vi "_shapiro2.vi"(0 "Bias_LO_equip":T4={"Node address"=19, "CAN Interface"="CAN0", "Cartridge band"=10, "Slave Node in"={"Address"=19, "Serial Number"=[16, -88, -112, 75, 1, 8, 0, 24]}, "ObjHandle out"=93192256, "POL"=1, "sb"=1, "GPIB_SM (SIS S,V)"="24", "GPIB_DMM (SIS I)"="22", "GPIB_SM (MAG I) "="25", "GPIB_SG(LO)"="19", "GPIB_PW (PAMP) "="6", "GPIB_TMP1(8ch)"="12", "GPIB_TMP2(2ch)  "="13", "WCA_avg"=10, "Rsen"=10.0, "BiasModule"=1, "LOModule "=2, "WCA_LO_FREQ_SET"={"YTO Low freq. [GHz]"=14.66, "YTO High freq. [GHz]"=17.5, "Kvco"=1, "Lock Pol."=0, "SET LO FREQ"=104.0, "Multiplier"=6.0, "YTO (HEX)"=3847, "YTO coarse( FREQ)"=17.328005, "NULL PLL INTEGRATOR"=FALSE}, "Res for"=0} {"Res for" items=["none", "series res", "parallel res"]; "WCA_LO_FREQ_SET"."YTO coarse( FREQ)" min=25 max=150 step=0.0001 format="%.3f"; "WCA_LO_FREQ_SET"."Multiplier" min=3 max=6 step=3; "WCA_LO_FREQ_SET"."SET LO FREQ" min=25 max=150 step=0.0001 format="%.3f"; "WCA_LO_FREQ_SET"."Lock Pol." items=["Lower", "Upper"]; "WCA_LO_FREQ_SET"."Kvco" items=["7.5MHz/V", "15MHz/V"]; "WCA_LO_FREQ_SET"."YTO High freq. [GHz]" format="%.3f"; "WCA_LO_FREQ_SET"."YTO Low freq. [GHz]" format="%.3f"; "LOModule" items=["Manual Gunn+PAMP"=0, "B10Lab LO"=1, "WCA LO"=2, ""=3, "YIG発信器"=4, "none"=99]; "BiasModule" items=["B10Lab Bias"=0, "WCA BiasModule"=1, "none"=99]; "Slave Node in"."Serial Number" format="%.0x"; "Slave Node in"."Address" format="%.0x"; "Cartridge band" max=10 step=1; "Node address" format="%.0x"}, 1 "Control":T2={"GPIB_ATT"="28", "6501Dev#"=1, "GPIB_SP"="18", "GPIB_PM"="13", "GPIB_DSA"="11", "GPIB_DMM (TPD)"="23", "GPIB_MPI"="COM5", "mortor設定"=[{"Axis"=0, "ID"=0, "HIspeed"=200.0, "LOspeed"=100.0, "ACCEL(ms)"=100.0, "Sratio"=50.0, "フリーラン\n"=FALSE, "文字列"="DSB HOT/COLD"}, {"Axis"=1, "ID"=0, "HIspeed"=4.0, "LOspeed"=4.0, "ACCEL(ms)"=100.0, "Sratio"=50.0, "フリーラン\n"=TRUE, "文字列"="SubMM Att"}, {"Axis"=0, "ID"=0, "HIspeed"=200.0, "LOspeed"=100.0, "ACCEL(ms)"=100.0, "Sratio"=50.0, "フリーラン\n"=FALSE, "文字列"="MPI Port1"}, {"Axis"=1, "ID"=0, "HIspeed"=200.0, "LOspeed"=100.0, "ACCEL(ms)"=100.0, "Sratio"=50.0, "フリーラン\n"=FALSE, "文字列"="MPI Port2"}, {"Axis"=1, "ID"=0, "HIspeed"=200.0, "LOspeed"=100.0, "ACCEL(ms)"=100.0, "Sratio"=50.0, "フリーラン\n"=TRUE, "文字列"="gainComp"}], "DATAパス"=path "L:/cartridge/assembly/SN03/03-13/110627_GUNNDSB_full_P0", "DBパス "=path "Z:/band10/Labview_ALMA/MIX95/test", "comment"="110627_gunndsbfull_P0", "ColdCarts"="003601", "Th"=299.0, "Tc"=83.0, "Set_SIS_volt"=2.1774193548387095, "Offset"=0.0, "control"=0, "FreqLO"=936.0, "Set_Mag_Cur"=9.671532846715328, "MPI offset(mm)"=23.166, "HOT/COLD"=0} {"HOT/COLD" items=["DSB", "SBR", "GainComp"]; "control" items=["CLOSE LOOP", "OPEN LOOP", "Not Control"]}, 2 "shapiro":T5={"start(mA)"=7.5, "stop(mA)"=12.5, "step(mA)"=0.1, "start(mV)"=1.2, "stop(mV)"=2.4, "step(mV)"=0.05, "file_name"="", "パス"=path "", "save?"=FALSE}, 3 "demag":T1={"Start(mA)"=50.0, "Time(ms)"=200.0, "step"=1.0}) -> (7 "min Mag current":dbl=9.299999999999994)   [LabVIEW 2017]
uses:
  __sub_vi/WCA_NAOJ_sub_vi/WCA_Global.vi
  <vilib>/express/express arith-compare/Formula/XNode/ExpressFormulaBlockNode.xnode
panel:
  out "setV  2":dbl=2.0500000000000003 format="%^#_3e"
  out "read V 2":dbl=1.9895172119140625
  out "read V":dbl=1.9895172119140625
  out "setV":dbl=2.0500000000000003 format="%^#_3e"
  in  "Time1":i32=1000
  in  "time0":i32=1000
  in  "set0?":bool=TRUE
  out "最終ｖ－P":cluster{"配列":dbl[], "配列 2":dbl[]}(graph)={"配列"=[1.1456298828125, 1.192474365234375, 1.2392425537109375, 1.2921142578125, 1.3437652587890625, 1.3919830322265625, 1.4446258544921875, 1.498565673828125, 1.551055908203125, 1.5949249267578125, 1.641693115234375, 1.691741943359375, 1.7388916015625, 1.7914581298828125, 1.841278076171875, 1.8906402587890625, 1.94244384765625, 1.9892120361328125, 2.0401763916015625, 2.0946502685546875, 2.142181396484375, 2.1912384033203125, 2.2409820556640625, 2.299041748046875, 2.3421478271484375], "配列 2"=[-30.6280724, -30.7126453, -30.6432113, -29.8285878, -28.8226745, -28.2742312, -27.7713224, -27.416188, -27.2844051, -27.2606276, -27.1514704, -26.9669342, -26.9316475, -26.9688126, -26.6291899, -25.4204539, -27.5721648, -25.6077726, -26.8063028, -27.3817095, -27.5837271, -27.7222411, -27.8415536, -28.2694503, -28.7533358]}
  out "error out":errorcluster caption="エラー出力"
  out "Link済み":bool=TRUE
  in  "i-vクラスタ":T3={"start(mV)"=1.2, "stop(mV)"=2.4, "step(mV)"=0.05, "file_name"="", "IF OFF/ON"=TRUE, "SAVE OFF/ON"=FALSE, "frq(GHz)"=8.0, "avg"=1, "Sweep回数 "=0, "VminfromSS"=0.05, "測定モード"=1, "V　opt"=0} {"測定モード" items=["電圧スイープ", "毎回HOT/COLD"]; "Sweep回数" items=["一回のみ", "Hot/Cold"]}
  out "初期値のV-P":cluster{dbl[], dbl[]}(graph)={[1.144561767578125, 1.1879730224609375, 1.2427520751953125, 1.2915802001953125, 1.34521484375, 1.3924407958984375, 1.4434051513671875, 1.4994049072265625, 1.5497589111328125, 1.5975189208984375, 1.6425323486328125, 1.693572998046875, 1.742706298828125, 1.7903900146484375, 1.838531494140625, 1.8914031982421875, 1.933746337890625, 1.9895172119140625, 2.041778564453125, 2.09136962890625, 2.1396636962890625, 2.1887969970703125, 2.2403717041015625, 2.2969818115234375, 2.3427581787109375], [-30.8304151, -30.6772316, -30.107581, -29.8432144, -27.7399153, -28.1617408, -27.8889748, -27.5394179, -26.7829628, -26.8468134, -26.4610859, -24.7404096, -23.8501166, -23.4218326, -23.1909815, -22.4041456, -26.7635773, -19.9675096, -20.681012, -21.9305003, -23.9269468, -27.6053273, -27.9912893, -28.0575443, -28.1897034]}
  out "min":dbl=-25.2940201 format="%^#_3e"
  out "Imag　vs P":cluster{dbl[], dbl[]}(graph)={[7.5, 7.6, 7.699999999999999, 7.799999999999999, 7.899999999999999, 7.999999999999998, 8.099999999999998, 8.199999999999998, 8.299999999999997, 8.399999999999997, 8.499999999999996, 8.599999999999996, 8.699999999999996, 8.799999999999995, 8.899999999999995, 8.999999999999995, 9.099999999999994, 9.199999999999994, 9.299999999999994, 9.399999999999993, 9.499999999999993, 9.599999999999993, 9.699999999999992, 9.799999999999992, 9.899999999999991, 9.999999999999991, 10.09999999999999, 10.19999999999999, 10.29999999999999, 10.39999999999999, 10.49999999999999, 10.599999999999989, 10.699999999999989, 10.799999999999988, 10.899999999999988, 10.999999999999988, 11.099999999999987, 11.199999999999987, 11.299999999999986, 11.399999999999986, 11.499999999999986, 11.599999999999985, 11.699999999999985, 11.799999999999985, 11.899999999999984, 11.999999999999984, 12.099999999999984, 12.199999999999983, 12.299999999999983, 12.399999999999983, 12.499999999999982], [-19.9638353, -20.1224192, -20.3203745, -20.461387, -20.6775476, -20.8219024, -20.9481227, -21.0140396, -21.0412557, -21.0582317, -21.1095669, -21.1470253, -21.2842083, -21.6610961, -22.0660132, -22.772983, -23.7101758, -24.7300495, -25.2940201, -24.7962579, -23.8748733, -22.8188748, -21.9031444, -21.2534559, -20.9269821, -20.7228013, -20.6284768, -20.5521107, -20.5344835, -20.5554763, -20.5479088, -20.6079808, -20.6594033, -20.7001155, -20.7420899, -20.7889111, -20.8004769, -20.844337, -20.9141659, -20.907771, -20.9407614, -20.9712207, -21.005632, -21.0478521, -21.0781252, -21.2327487, -21.243586, -21.3534511, -21.5174431, -21.7408682, -21.9673929]}
  # "LO freq. [GHz]"
  # "YTO LOW\n/High Freq."
  # "ZERO Intgrtr"
  # "Node Address"
  # "Serial Number"
  # "Magnet current"
  # "SIS Bias range"
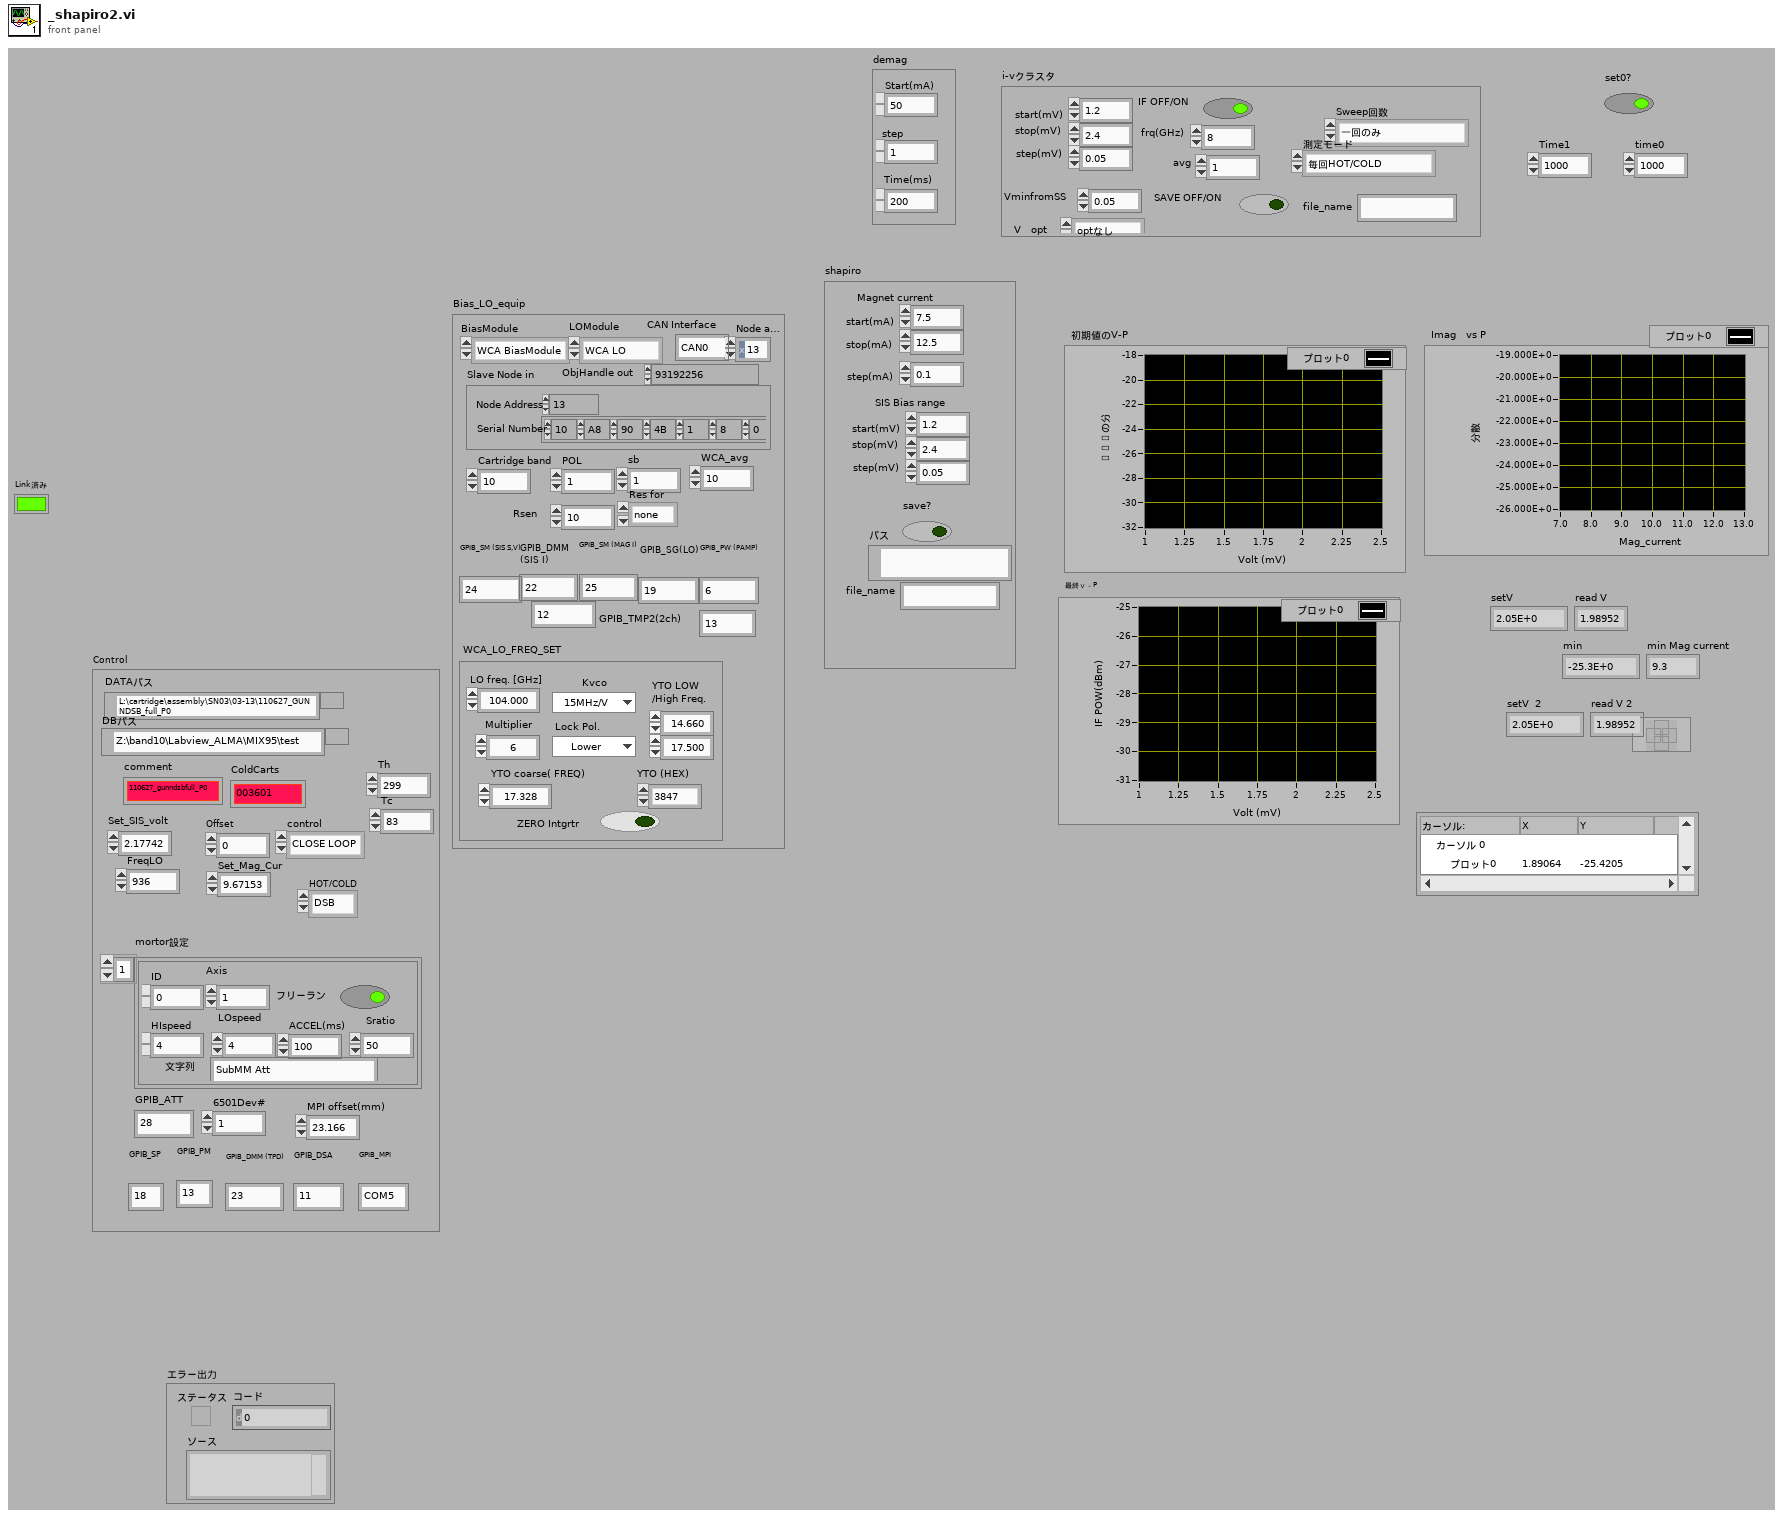
[diagram p1: front panel]
types:
  T1 = cluster{"Start(mA)":dbl, "Time(ms)":dbl, "step":dbl}
  T2 = cluster{"GPIB_ATT":string, "6501Dev#":i16, "GPIB_SP":string, "GPIB_PM":string, "GPIB_DSA":string, "GPIB_DMM (TPD)":string, "GPIB_MPI":string, "mortor設定":cluster{"Axis":i16, "ID":i16, "HIspeed":dbl, "LOspeed":dbl, "ACCEL(ms)":dbl, "Sratio":dbl, "フリーラン\n":bool, "文字列":string}[], "DATAパス":path, "DBパス ":path, "comment":string, "ColdCarts":string, "Th":dbl, "Tc":dbl, "Set_SIS_volt":dbl, "Offset":dbl, "control":u16, "FreqLO":dbl, "Set_Mag_Cur":dbl, "MPI offset(mm)":dbl, "HOT/COLD":u16}
  T3 = cluster{"start(mV)":dbl, "stop(mV)":dbl, "step(mV)":dbl, "file_name":string, "IF OFF/ON":bool, "SAVE OFF/ON":bool, "frq(GHz)":dbl, "avg":i32, "Sweep回数 ":u16, "VminfromSS":dbl, "測定モード":u16, "V　opt":u16}
  T4 = cluster{"Node address":u16, "CAN Interface":string, "Cartridge band":u32, "Slave Node in":cluster{"Address":i16, "Serial Number":i8[]}, "ObjHandle out":u32, "POL":u32, "sb":u32, "GPIB_SM (SIS S,V)":string, "GPIB_DMM (SIS I)":string, "GPIB_SM (MAG I) ":string, "GPIB_SG(LO)":string, "GPIB_PW (PAMP) ":string, "GPIB_TMP1(8ch)":string, "GPIB_TMP2(2ch)  ":string, "WCA_avg":i32, "Rsen":dbl, "BiasModule":u16, "LOModule ":u16, "WCA_LO_FREQ_SET":cluster{"YTO Low freq. [GHz]":sgl, "YTO High freq. [GHz]":sgl, "Kvco":u16, "Lock Pol.":u16, "SET LO FREQ":sgl, "Multiplier":sgl, "YTO (HEX)":u16, "YTO coarse( FREQ)":sgl, "NULL PLL INTEGRATOR":bool}, "Res for":u16}
  T5 = cluster{"start(mA)":dbl, "stop(mA)":dbl, "step(mA)":dbl, "start(mV)":dbl, "stop(mV)":dbl, "step(mV)":dbl, "file_name":string, "パス":path, "save?":bool}
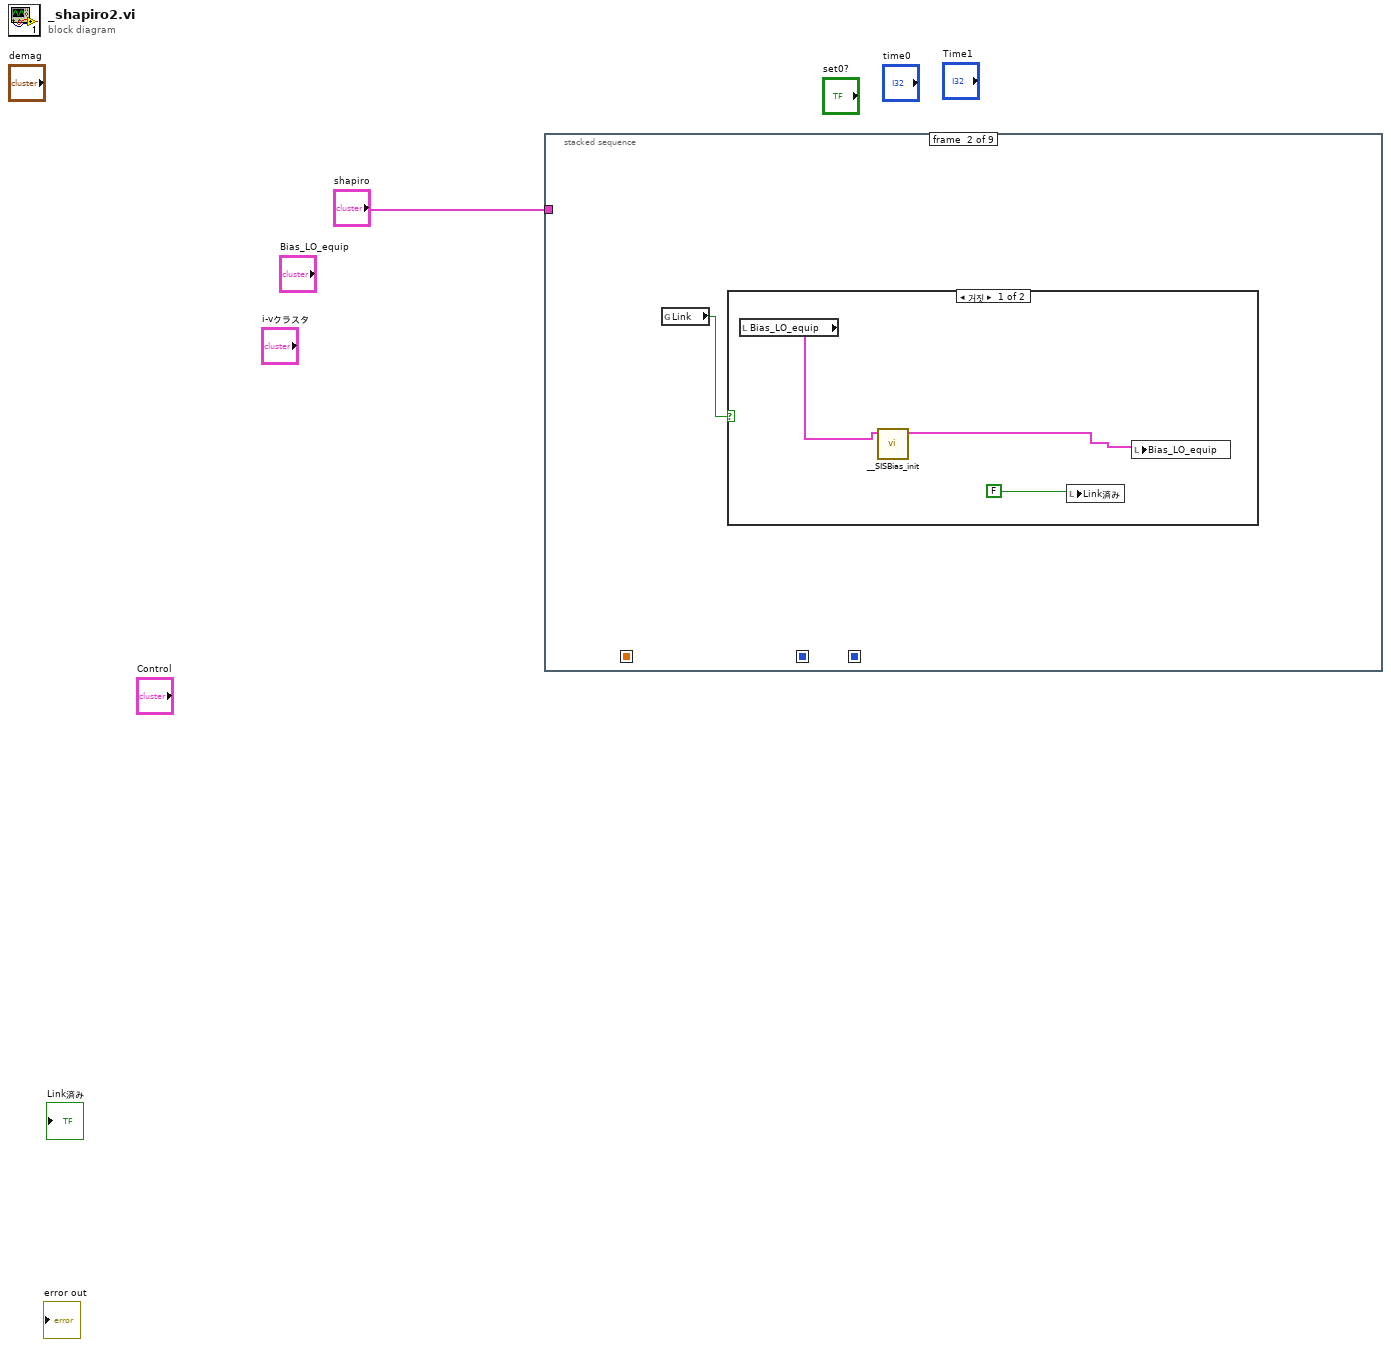
[diagram p0: block diagram]
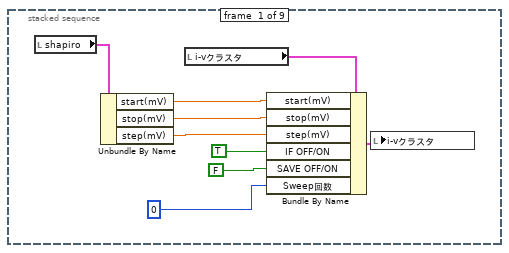
[diagram p2: hidden frame]
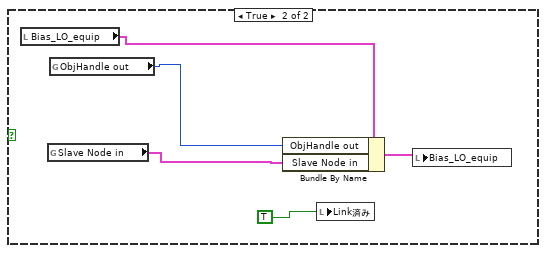
[diagram p3: hidden frame]
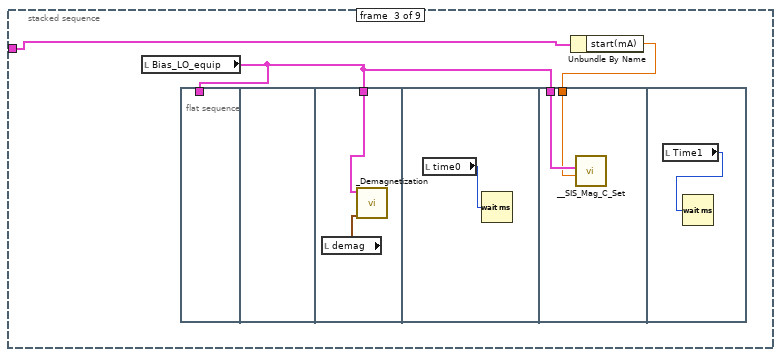
[diagram p4: hidden frame]
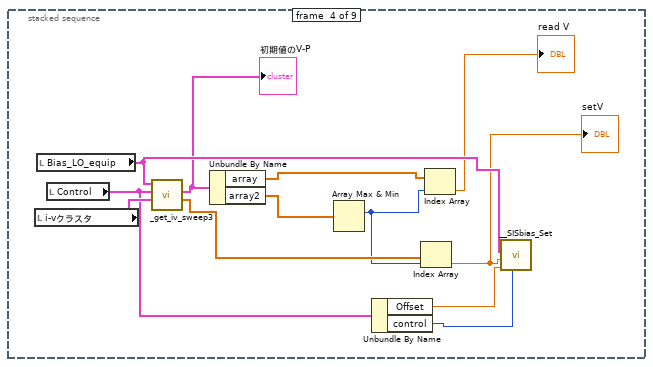
[diagram p5: hidden frame]
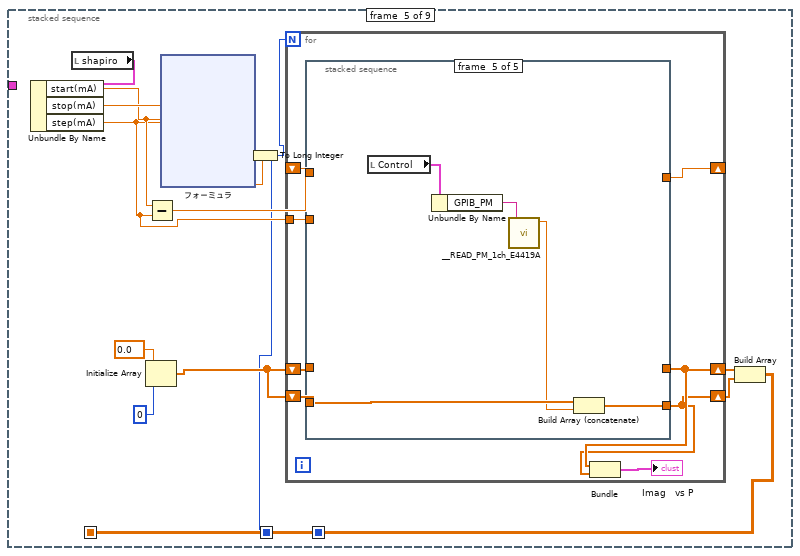
[diagram p6: hidden frame]
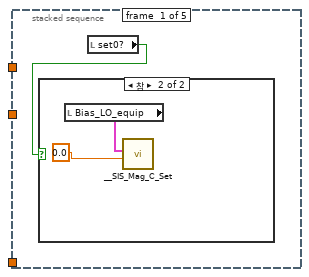
[diagram p7: hidden frame]
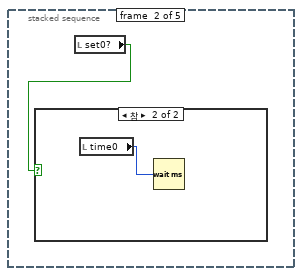
[diagram p9: hidden frame]
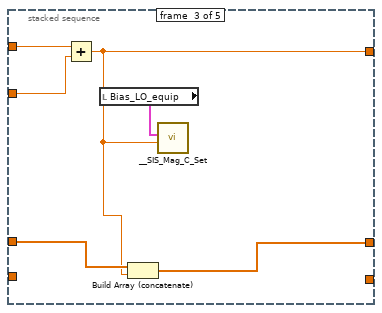
[diagram p11: hidden frame]
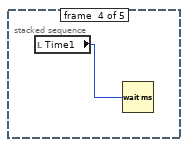
[diagram p12: hidden frame]
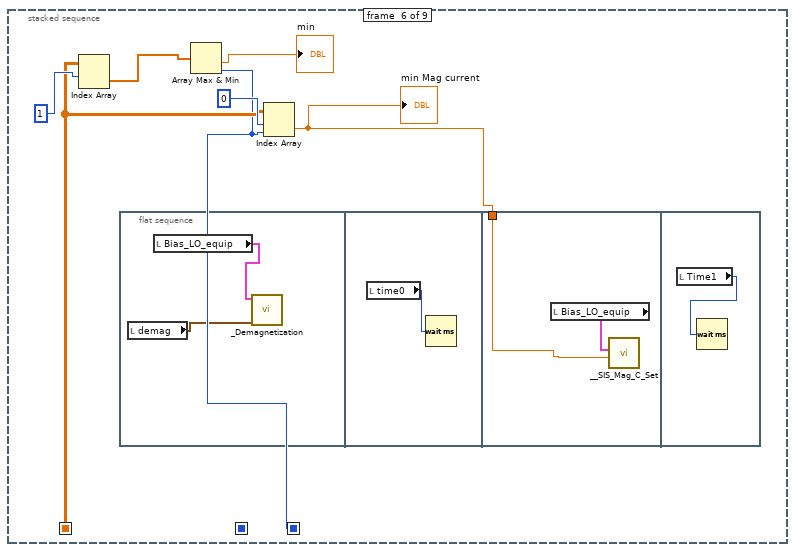
[diagram p13: hidden frame]
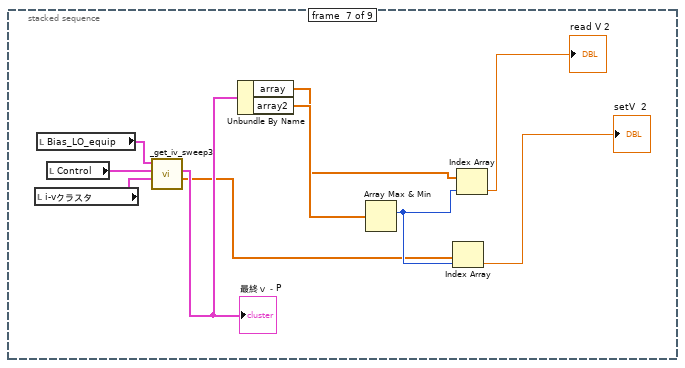
[diagram p14: hidden frame]
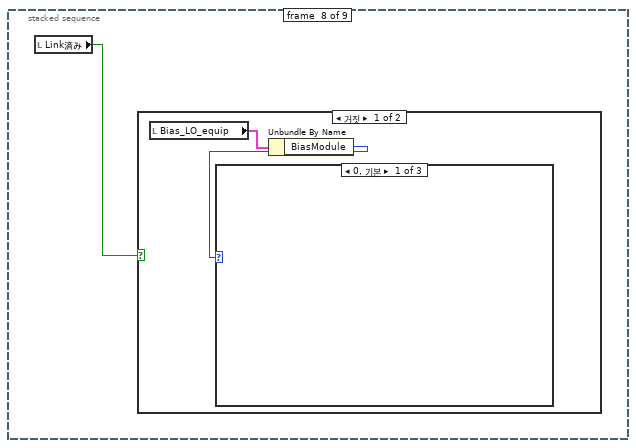
[diagram p15: hidden frame]
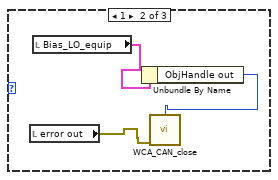
[diagram p16: hidden frame]
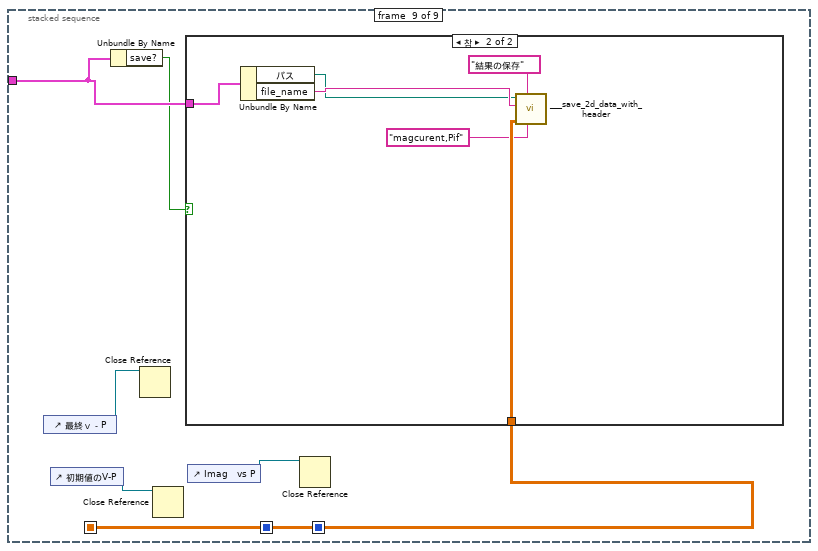
[diagram p19: hidden frame]
diagram:
  n1 = stacked-sequence {
    seq-local: [_ _ _ _ w42 _ _ _ _] -> [_ _ _ _ _ w93 _ _ w125]
    seq-local: [_ _ _ _ w41 _ _ _ _] -> [_ _ _ _ _ _ _ _ _]
    seq-local: [_ _ _ _ _ w92 _ _ _] -> [_ _ _ _ _ _ _ _ _]
    tunnel: "shapiro" -> [_ _ w22 _ _ _ _ _ w124]
    frame #0 {
      n2 = local read "shapiro"() -> (w10:T5)
      n3 = Unbundle By Name(w10) -> ("start(mV)"=w8:dbl, "stop(mV)"=w7:dbl, "step(mV)"=w6:dbl)
      n4 = local read "i-vクラスタ"() -> (w9:T3)
      n5 = Bundle By Name(cluster=w9, "start(mV)"=w8, "stop(mV)"=w7, "step(mV)"=w6, "IF OFF/ON"=TRUE, "SAVE OFF/ON"=FALSE, "Sweep回数"=0) -> (w3:T3)
      n6 = local write "i-vクラスタ"(w3) -> ()
    }
    frame #1 {
      n7 = global read "WCA_Global.vi" "Link"() -> (w11:bool)
      n8 = case shown="거짓" w11 {
        frame False {
          n9 = local read "Bias_LO_equip"() -> (w13:T4)
          n10 = call "__SISBias_init.vi"("Bias_LO_equip"=w13) -> ("Bias_LO_equip 2"=w12:T4)  [unwired: 4 in, 2 out]
          n11 = local write "Link済み"(FALSE) -> ()
          n12 = local write "Bias_LO_equip"(w12) -> ()
        }
        frame True {
          n13 = local read "Bias_LO_equip"() -> (w18:T4)
          n14 = global read "WCA_Global.vi" "Slave Node in"() -> (w16:cluster{"Address":i16, "Serial Number":i8[]})
          n15 = global read "WCA_Global.vi" "ObjHandle out"() -> (w17:u32)
          n16 = Bundle By Name(cluster=w18, "ObjHandle out"=w17, "Slave Node in"=w16) -> (w19:T4)
          n17 = local write "Link済み"(TRUE) -> ()
          n18 = local write "Bias_LO_equip"(w19) -> ()
        }
      }
    }
    frame #2 {
      n19 = local read "Bias_LO_equip"() -> (w20:T4)
      n20 = flat-sequence {
        tunnel: w20 -> [_]
        tunnel: w20 -> [w23]
        tunnel: w20 -> [w27]
        tunnel: w21 -> [w26]
        frame #0 {
        }
        frame #1 {
        }
        frame #2 {
          n21 = local read "demag"() -> (w24:T1)
          n22 = call "_Demagnetization.vi"("demag"=w24, "Bias_LO_equip"=w23) -> ()  [unwired: 10 in]
        }
        frame #3 {
          n23 = local read "time0"() -> (w25:i32)
          n24 = Wait (ms)(milliseconds to wait=w25) -> ()  [unwired: 1 out]
        }
        frame #4 {
          n25 = call "__SIS_Mag_C_Set.vi"("Set_Mag_C"=w26, "Bias_LO_equip"=w27) -> ()  [unwired: 10 in]
        }
        frame #5 {
          n26 = local read "Time1"() -> (w28:i32)
          n27 = Wait (ms)(milliseconds to wait=w28) -> ()  [unwired: 1 out]
        }
      }
      n28 = Unbundle By Name(w22) -> ("start(mA)"=w21:dbl)
    }
    frame #3 {
      n29 = local read "i-vクラスタ"() -> (w40:T3)
      n30 = local read "Bias_LO_equip"() -> (w37:T4)
      n31 = local read "Control"() -> (w36:T2)
      n32 = call "_get_iv_sweep3.vi"("I-V class"=w40, "Control"=w36, "Bias_LO_equip"=w37) -> ("Vset"=w38:dbl[], "VP class"=w33:cluster{"array":dbl[], "array2":dbl[]})  [unwired: 2 in, 1 out]
      "初期値のV-P" <- w33
      n33 = Unbundle By Name(w33) -> ("array"=w31:dbl[], "array2"=w39:dbl[])
      n34 = Array Max & Min(array=w39) -> (max index (indices)=w30:i32)  [unwired: 3 out]
      n35 = Unbundle By Name(w36) -> ("Offset"=w35:dbl, "control"=w34:u16)
      n36 = Index Array(array=w38, index=w30) -> (element=w32:dbl)
      "setV" <- w32
      n37 = Index Array(array=w31, index=w30) -> (element=→"read V":dbl)
      n38 = call "__SISbias_Set.vi"("SIS　Mode"=w34, "Offset"=w35, "Set_V"=w32, "Bias_LO_equip"=w37) -> ()  [unwired: 7 in, 1 out]
    }
    frame #4 {
      n39 = local read "shapiro"() -> (w53:T5)
      n40 = Unbundle By Name(w53) -> ("start(mA)"=w50:dbl, "stop(mA)"=w52:dbl, "step(mA)"=w48:dbl)
      n41 = Initialize Array(0.0, 0) -> (w45:dbl[])
      n42 = Subtract(x=w50, y=w48) -> (x-y=w49:dbl)
      n43 = xnode "フォーミュラ"("start"=w50, "stop"=w52, "step"=w48) -> ("結果"=w51:dbl)  [unwired: 1 in, 1 out]
      n44 = To Long Integer(number=w51) -> (32bit integer=w41:i32)
      n45 = for {
        N: w41 -> [_]
        shift-right: [w71] -> _
        shift-left: w49 -> [w73]
        tunnel: w48 -> [w72]
        shift-right: [w67] -> w44
        shift-left: w45 -> [w70]
        shift-right: [w66] -> w43
        shift-left: w45 -> [w69]
        n46 = stacked-sequence {
          tunnel: w73 -> [_ _ w84 _ _]
          tunnel: w72 -> [_ _ w83 _ _]
          tunnel: [_ _ w80 _ _] -> w71
          tunnel: w70 -> [_ _ w82 _ _]
          tunnel: [_ _ w81 _ _] -> w67
          tunnel: w69 -> [_ _ _ _ w90]
          tunnel: [_ _ _ _ w89] -> w66
          frame #0 {
            n47 = local read "set0?"() -> (w74:bool)
            n48 = case shown="참" w74 {
              frame False {
              }
              frame True {
                n49 = local read "Bias_LO_equip"() -> (w75:T4)
                n50 = call "__SIS_Mag_C_Set.vi"("Set_Mag_C"=0.0, "Bias_LO_equip"=w75) -> ()  [unwired: 10 in]
              }
            }
          }
          frame #1 {
            n51 = local read "set0?"() -> (w77:bool)
            n52 = case shown="참" w77 {
              frame False {
              }
              frame True {
                n53 = local read "time0"() -> (w78:i32)
                n54 = Wait (ms)(milliseconds to wait=w78) -> ()  [unwired: 1 out]
              }
            }
          }
          frame #2 {
            n55 = Add(x=w84, y=w83) -> (x+y=w80:dbl)
            n56 = local read "Bias_LO_equip"() -> (w79:T4)
            n57 = Build Array (concatenate)(w82, w80) -> (w81:dbl[])
            n58 = call "__SIS_Mag_C_Set.vi"("Set_Mag_C"=w80, "Bias_LO_equip"=w79) -> ()  [unwired: 10 in]
          }
          frame #3 {
            n59 = local read "Time1"() -> (w85:i32)
            n60 = Wait (ms)(milliseconds to wait=w85) -> ()  [unwired: 1 out]
          }
          frame #4 {
            n61 = local read "Control"() -> (w86:T2)
            n62 = Unbundle By Name(w86) -> ("GPIB_PM"=w87:string)
            n63 = call "__READ_PM_1ch_E4419A.VI"("GPIB"=w87) -> ("chA"=w88:dbl)  [unwired: 6 in]
            n64 = Build Array (concatenate)(w90, w88) -> (w89:dbl[])
          }
        }
        n65 = Bundle(w67, w66) -> (→"Imag　vs P":cluster{dbl[], dbl[]})  [unwired: 1 in]
      }
      n66 = Build Array(w44, w43) -> (w42:dbl[][])
    }
    frame #5 {
      n67 = Index Array(array=w93, index (row)=1) -> (element=w96:dbl[])  [unwired: 1 in]
      n68 = flat-sequence {
        tunnel: w91 -> [w101]
        frame #0 {
          n69 = local read "demag"() -> (w98:T1)
          n70 = local read "Bias_LO_equip"() -> (w99:T4)
          n71 = call "_Demagnetization.vi"("demag"=w98, "Bias_LO_equip"=w99) -> ()  [unwired: 10 in]
        }
        frame #1 {
          n72 = local read "time0"() -> (w100:i32)
          n73 = Wait (ms)(milliseconds to wait=w100) -> ()  [unwired: 1 out]
        }
        frame #2 {
          n74 = local read "Bias_LO_equip"() -> (w102:T4)
          n75 = call "__SIS_Mag_C_Set.vi"("Set_Mag_C"=w101, "Bias_LO_equip"=w102) -> ()  [unwired: 10 in]
        }
        frame #3 {
          n76 = local read "Time1"() -> (w103:i32)
          n77 = Wait (ms)(milliseconds to wait=w103) -> ()  [unwired: 1 out]
        }
      }
      n78 = Array Max & Min(array=w96) -> (min value=→"min":dbl, min index (indices)=w92:i32)  [unwired: 2 out]
      n79 = Index Array(array=w93, index (row)=0, index (col)=w92) -> (element=w91:dbl)
      "min Mag current" <- w91
    }
    frame #6 {
      n80 = local read "i-vクラスタ"() -> (w111:T3)
      n81 = local read "Bias_LO_equip"() -> (w113:T4)
      n82 = local read "Control"() -> (w112:T2)
      n83 = call "_get_iv_sweep3.vi"("I-V class"=w111, "Control"=w112, "Bias_LO_equip"=w113) -> ("Vset"=w104:dbl[], "VP class"=w105:cluster{"array":dbl[], "array2":dbl[]})  [unwired: 2 in, 1 out]
      "最終ｖ－P" <- w105
      n84 = Unbundle By Name(w105) -> ("array"=w108:dbl[], "array2"=w110:dbl[])
      n85 = Array Max & Min(array=w110) -> (max index (indices)=w107:i32)  [unwired: 3 out]
      n86 = Index Array(array=w104, index=w107) -> (element=→"setV  2":dbl)
      n87 = Index Array(array=w108, index=w107) -> (element=→"read V 2":dbl)
    }
    frame #7 {
      n88 = local read "Link済み"() -> (w114:bool)
      n89 = case shown="거짓" w114 {
        frame False {
          n90 = local read "Bias_LO_equip"() -> (w116:T4)
          n91 = Unbundle By Name(w116) -> ("BiasModule"=w115:u16)
          n92 = case shown="0, 기본" w115 {
            frame 0, Default {
            }
            frame 1 {
              n93 = local read "error out"() -> (w119:errorcluster)
              n94 = local read "Bias_LO_equip"() -> (w118:T4)
              n95 = Unbundle By Name(w118) -> ("ObjHandle out"=w117:u32)
              n96 = call "WCA_CAN_close.vi"("ObjHandle in"=w117, "error in (no error)"=w119) -> ()  [unwired: 13 in, 1 out]
            }
            frame 99 {
            }
          }
        }
        frame True {
        }
      }
    }
    frame #8 {
      n97 = control-ref of="最終ｖ－P"() -> (w120:refnum<vi>)
      n98 = control-ref of="初期値のV-P"() -> (w121:refnum<vi>)
      n99 = Unbundle By Name(w124) -> ("save?"=w123:bool)
      n100 = Close Reference(reference=w120) -> ()  [unwired: 1 in, 1 out]
      n101 = Close Reference(reference=w121) -> ()  [unwired: 1 in, 1 out]
      n102 = case shown="참" w123 {
        tunnel: w125 -> [_ w130]
        tunnel: w124 -> [_ w127]
        frame False {
        }
        frame True {
          n103 = Unbundle By Name(w127) -> ("パス"=w129:path, "file_name"=w131:string)
          n104 = call "___save_2d_data_with_header.vi"("ヘッダー"="magcurent,Pif", "プロンプト"="結果の保存", "配列"=w130, "file_name"=w131, "パス"=w129) -> ()  [unwired: 6 in, 1 out]
        }
      }
      n105 = control-ref of="Imag　vs P"() -> (w122:refnum<vi>)
      n106 = Close Reference(reference=w122) -> ()  [unwired: 1 in, 1 out]
    }
  }
